vi "PRIME Telescope Move To RA and DEC.vi"(8 "error in (no error)":errorcluster, 10 "Object":T1, 11 "connection ID":refnum<k5>) -> (0 "error out":errorcluster, 3 "connection ID dup":refnum<k5>)   [LabVIEW 2024, in "PRIME Telescope.lvclass"]
uses:
  PRIME Telescope.lvclass
  typedefs/CC cluster Object.ctl
  typedefs/CC cluster sidereal rate.ctl
  typedefs/CC cluster RA and DEC.ctl
  typedefs/cc cluster muRA muDEC.ctl
  CC cluster Telescope Offsets.ctl
  Telescope cluster Equinox.ctl
  Telescope cluster Parallax.ctl
  Telescope cluster Rotator.ctl
  Telesope ring Frame.ctl
  Telescope.lvclass
panel:
  out "resulting string":string
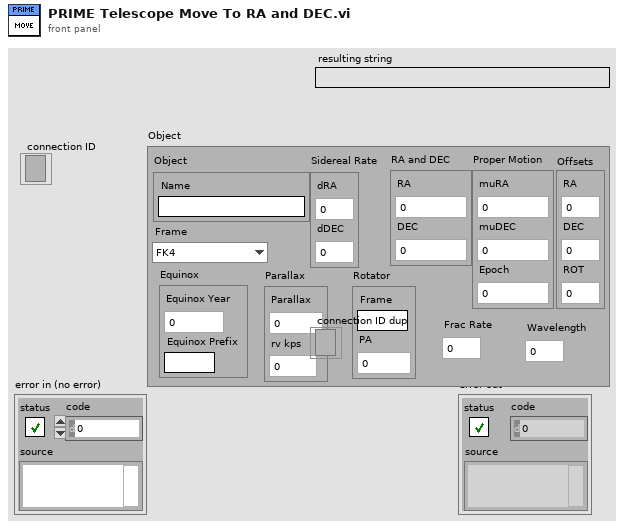
[diagram p1: front panel]
types:
  T1 = typedef "CC cluster Object.ctl" = cluster{"Object":cluster{"Name":string}, "Sidereal Rate":T2, "RA and DEC":T3, "Proper Motion":T4, "Offsets":T5, "Equinox":T6, "Parallax":T7, "Rotator":T8, "Frame":T9, "Frac Rate":dbl, "Wavelength":dbl}
  T2 = typedef "CC cluster sidereal rate.ctl" = cluster{"dRA":dbl, "dDEC":dbl}
  T3 = typedef "CC cluster RA and DEC.ctl" = cluster{"RA":dbl, "DEC":dbl}
  T4 = typedef "cc cluster muRA muDEC.ctl" = cluster{"muRA":dbl, "muDEC":dbl, "Epoch":dbl}
  T5 = typedef "CC cluster Telescope Offsets.ctl" = cluster{"RA":dbl, "DEC":dbl, "ROT":dbl}
  T6 = typedef "Telescope cluster Equinox.ctl" = cluster{"Equinox Year":i32, "Equinox Prefix":string}
  T7 = typedef "Telescope cluster Parallax.ctl" = cluster{"Parallax":dbl, "rv kps":dbl}
  T8 = typedef "Telescope cluster Rotator.ctl" = cluster{"Frame":string, "PA":dbl}
  T9 = typedef "Telesope ring Frame.ctl" = enum16{"FK4", "FK5", "APPT", "GAPPT", "AZEL"}
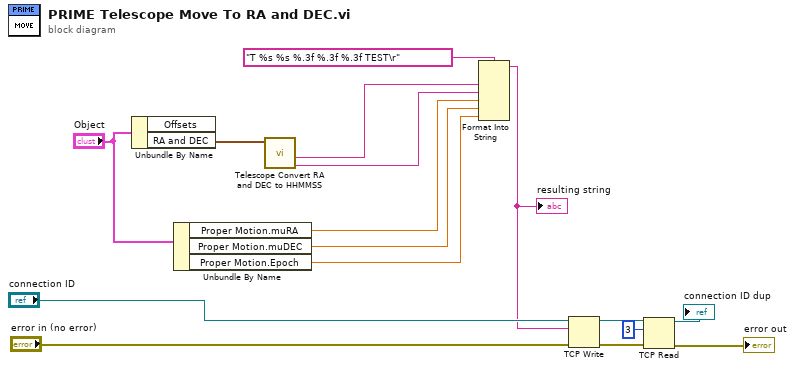
[diagram p0: block diagram]
diagram:
  n1 = Unbundle By Name("Object") -> ("RA and DEC"=w3:T3)  [unwired: 1 out]
  n2 = Unbundle By Name("Object") -> ("Proper Motion.muRA"=w8:dbl, "Proper Motion.muDEC"=w7:dbl, "Proper Motion.Epoch"=w6:dbl)
  n3 = call "Telescope Convert RA and DEC to HHMMSS.vi"("RA and DEC"=w3) -> ("Dec String"=w4:string, "RA String"=w5:string)  [unwired: 7 in, 2 out]
  n4 = Format Into String(format string="T %s %s %.3f %.3f %.3f TEST\r", w5, w4, w8, w7, w6) -> (resulting string=w13:string)  [unwired: 2 in, 1 out]
  "resulting string" <- w13
  n5 = TCP Write(connection ID="connection ID", data in=w13, error in (no error)="error in (no error)") -> (connection ID out=w11:refnum<k5>, error out=w12:errorcluster)  [unwired: 1 in, 1 out]
  n6 = TCP Read(connection ID=w11, bytes to read=3, error in (no error)=w12) -> (connection ID out=→"connection ID dup":refnum<k5>, error out=→"error out":errorcluster)  [unwired: 2 in, 1 out]
